vi "Read Port Names.vi"(8 "error in (no error)":errorcluster, 11 "NICal5501 in":refnum<class "Cal Standard.lvclass">) -> (0 "error out":errorcluster, 2 "Port Names":string[](array[string]), 3 "NICal5501 out":refnum<class "Cal Standard.lvclass">)   [LabVIEW 2023, in "NI Cal-5501 Cal Standard.lvlib" / "Cal Standard.lvclass"]
uses:
  Cal Standard.lvclass
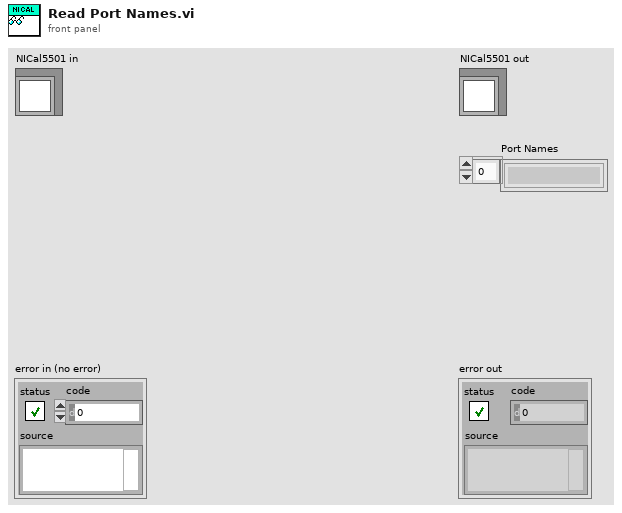
[diagram p1: front panel]
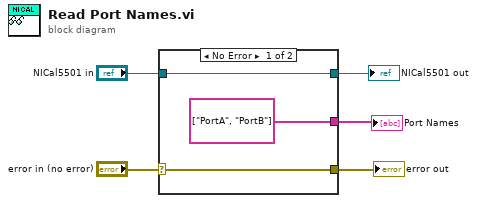
[diagram p0: block diagram]
diagram:
  n1 = case shown="No Error" "error in (no error)" {
    selector: "error in (no error)" -> [w8 w9]
    tunnel: [w8 w9] -> w1
    tunnel: [w7 w10] -> w4
    tunnel: "NICal5501 in" -> [w7 w10]
    tunnel: [string[] ["PortA", "PortB"] ("ACM4509 Port Names") _] -> w5
    frame No Error {
    }
    frame Error {
    }
  }
  "error out" <- w1
  "NICal5501 out" <- w4
  "Port Names" <- w5
